vi "17.-Curva Característica de Datos Muestreados.vi"() -> ()   [LabVIEW 2020]
uses:
  <vilib>/Analysis/baseanly.llb/Mean (DBL).vi
  <vilib>/Analysis/NI_AALPro.lvlib
  <vilib>/Analysis/NI_AALBase.lvlib
panel:
  out "Polynomial Coefficients":dbl[](array[numeric])
  out "Waveform Graph":T1(graph)
  out "Thermometer":dbl(slide) scale=0.0..100.0
  out "mean":dbl format="%0.2f"
  out "min value":dbl
  out "max value":dbl
  in  "polynomial order":i32=2
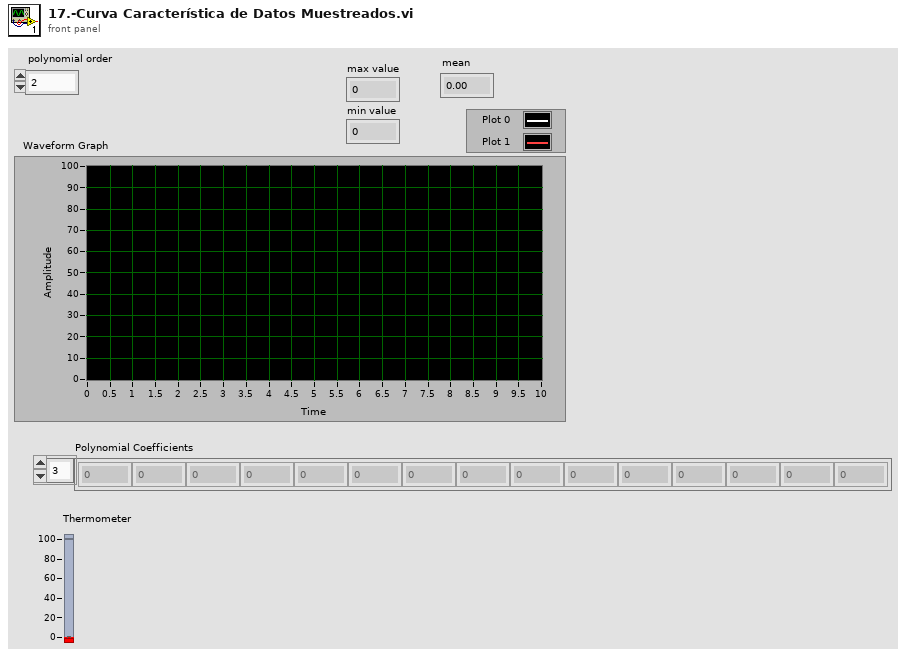
[diagram p1: front panel]
types:
  T1 = cluster{i32, "y":dbl, "Best Polynomial Fit":dbl[]}[]
  T2 = cluster{i32, "y":dbl, "Best Polynomial Fit":dbl[]}
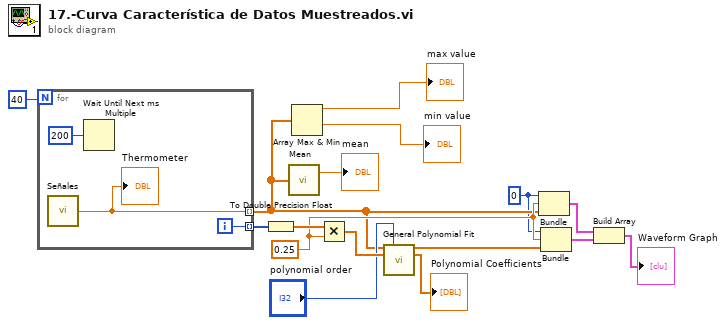
[diagram p0: block diagram]
diagram:
  w5 = 0
  w7 = 0.25 ("y")
  n1 = for {
    N: 40 -> [_]
    tunnel: [w17] -> w6 mode=indexing
    tunnel: [w18] -> w15 mode=indexing
    i -> [w18]
    n2 = call "Señales.vi"() -> ("Señal"=w17:dbl)
    "Thermometer" <- w17
    n3 = Wait Until Next ms Multiple(millisecond multiple=u32 200) -> ()  [unwired: 1 out]
  }
  n4 = To Double Precision Float(number=w15) -> (double precision float=w14:dbl[])
  n5 = call-poly <vilib>:"Mean.vi"("X"=w6) -> ("mean"=→"mean":dbl)  [unwired: 1 out]
  n6 = Array Max & Min(array=w6) -> (max value=→"max value":dbl, min value=→"min value":dbl)  [unwired: 2 out]
  n7 = Multiply(x=w14, y=w7) -> (x*y=w13:dbl[])
  n8 = call <vilib>:"General Polynomial Fit.vi"("Y"=w6, "polynomial order"="polynomial order", "X"=w13) -> ("Best Polynomial Fit"=w8:dbl[], "Polynomial Coefficients"=→"Polynomial Coefficients":dbl[])  [unwired: 9 in, 2 out]
  n9 = Bundle "Bundle"(w5, "y"=w7, w6) -> (w4:cluster{i32, "y":dbl, dbl[]})  [unwired: 1 in]
  n10 = Bundle(w5, "y"=w7, "Best Polynomial Fit"=w8) -> (w3:T2)  [unwired: 1 in]
  n11 = Build Array "Build Array"(w4, w3) -> (→"Waveform Graph":T1)
